vi "Read All Stderr.vi"(6 "Per Read Size":i32=1024 max=30000, 8 "Error In":errorcluster, 10 "Total Read Size":i32=1024, 11 "Channel In":refnum<class "Channel.lvclass">) -> (0 "Error Out":errorcluster, 2 "Data":u8[](array[numeric]), 3 "Channel Out":refnum<class "Channel.lvclass">)   [LabVIEW 2018, in "Toolkit.lvlib" / "Channel.lvclass"]
doc: "Reads binary data from the STDERR stream of a SSH channel represented by this Channel object in chunks, or blocks, until the total read size is reached. This VI should be used if the <B>Total Read Size</B> is greater than 30KB because of a hard-coded per-read maximum of 30KB defined in the libssh2 shared library."
uses:
  Channel.lvclass
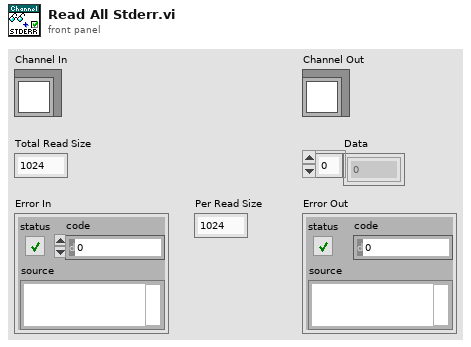
[diagram p1: front panel]
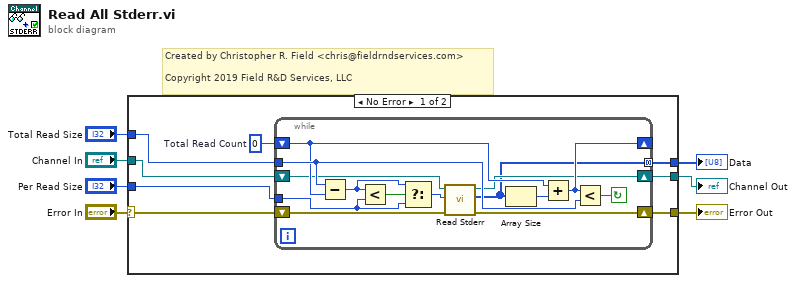
[diagram p0: block diagram]
diagram:
  # "Created by Christopher R. Field <chris@fieldrndservices.com>\n\nCopyright 2019 Field R&D Services, LLC"
  n1 = case shown="No Error" "Error In" {
    selector: "Error In" -> [w8 w30]
    tunnel: "Total Read Size" -> [w14 _]
    tunnel: "Per Read Size" -> [w13 _]
    tunnel: "Channel In" -> [w12 w31]
    tunnel: [w11 _] -> w4
    tunnel: [w10 w31] -> w3
    tunnel: [w9 w30] -> w2
    frame No Error {
      w15 = 0  # Total Read Count
      n2 = while {
        shift-right: [w20] -> w10
        shift-left: w12 -> [w17]
        shift-right: [w21] -> w9
        shift-left: w8 -> [w16]
        tunnel: [w19] -> w11 mode=concatenating
        shift-right: [w28] -> _
        shift-left: w15 -> [w25]
        tunnel: w14 -> [w26]
        tunnel: w13 -> [w22]
        stop <- w27 continue-if-true
        n3 = Subtract(x=w26, y=w25) -> (x-y=w23:i32)
        n4 = Less?(x=w23, y=w22) -> (x < y?=w24:bool)
        n5 = Select(t=w23, s=w24, f=w22) -> (s? t:f=w18:i32)
        n6 = call "Read Stderr.vi"("Error In"=w16, "Max Data Length"=w18, "Channel In"=w17) -> ("Error Out"=w21:errorcluster, "Data"=w19:u8[], "Channel Out"=w20:refnum<class "Channel.lvclass">)  [unwired: 6 in]
        n7 = Array Size(array=w19) -> (size(s)=w29:i32)
        n8 = Add(x=w25, y=w29) -> (x+y=w28:i32)
        n9 = Less?(x=w28, y=w26) -> (x < y?=w27:bool)
      }
    }
    frame Error {
    }
  }
  "Data" <- w4
  "Channel Out" <- w3
  "Error Out" <- w2
